vi "N Gaussians Fit Guess Parameters.vi"(8 "N":i32, 9 "Cursor X Array":dbl[](array[numeric]), 10 "Y Array":dbl[](array[numeric]), 11 "X Array":dbl[](array[numeric])) -> (1 "Guess Parameters Array":dbl[](array[numeric]), 2 "Y Array dup":dbl[](array[numeric]), 3 "X Array dup":dbl[](array[numeric]))   [LabVIEW 2019]
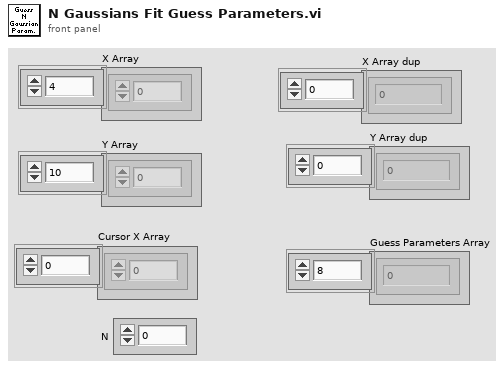
[diagram p1: front panel]
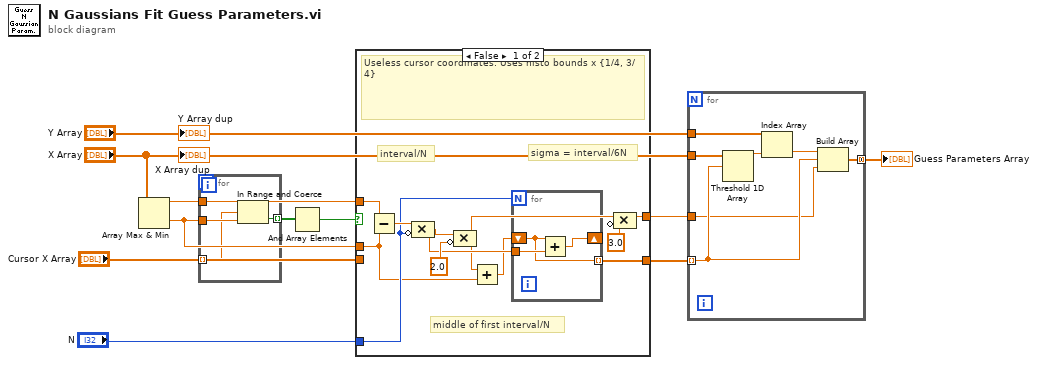
[diagram p0: block diagram]
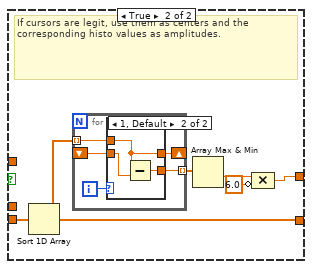
[diagram p2: hidden frame]
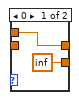
[diagram p3: hidden frame]
diagram:
  n1 = Array Max & Min(array="X Array") -> (max value=w4:dbl, min value=w3:dbl)  [unwired: 2 out]
  n2 = for {
    tunnel: w4 -> [w15]
    tunnel: w3 -> [w14]
    tunnel: "Cursor X Array" -> [w13] mode=indexing
    tunnel: [w12] -> w9 mode=indexing
    n3 = In Range and Coerce(upper limit=w15, x=w13, lower limit=w14) -> (In Range?=w12:bool)  [unwired: 1 out]
  }
  n4 = And Array Elements(Boolean array=w9) -> (logical AND=w1:bool)
  n5 = case shown="False" w1 {
    tunnel: "Cursor X Array" -> [_ w35]
    tunnel: [w21 w34] -> w7
    tunnel: [w20 w31] -> w5
    tunnel: w4 -> [w26 _]
    tunnel: w3 -> [w17 _]
    tunnel: "N" -> [w23 _]
    frame False {
      # "sigma = interval/6N"
      # "middle of first interval/N"
      # "interval/N"
      # "Useless cursor coordinates. Uses histo bounds x {1/4, 3/4}"
      n6 = Subtract(x=w26, y=w17) -> (x-y=w25:dbl)
      n7 = Compound Arithmetic op=MULTIPLY(w25, invert w23) -> (w22:dbl)
      n8 = Compound Arithmetic op=MULTIPLY(w22, invert 2.0 ("value")) -> (w18:dbl)
      n9 = Add(x=w18, y=w17) -> (x+y=w16:dbl)
      n10 = for {
        N: w23 -> [_]
        shift-right: [w29] -> _
        shift-left: w16 -> [w27]
        tunnel: w22 -> [w28]
        tunnel: [w27] -> w21 mode=indexing
        n11 = Add(x=w27, y=w28) -> (x+y=w29:dbl)
      }
      n12 = Compound Arithmetic op=MULTIPLY(w18, invert 3.0 ("value")) -> (w20:dbl)
    }
    frame True {
      # "If cursors are legit, use them as centers and the corresponding histo values as amplitudes."
      n13 = Sort 1D Array(array=w35) -> (sorted array=w34:dbl[])
      n14 = for {
        tunnel: w34 -> [w38] mode=indexing
        shift-right: [w39] -> _
        shift-left: _ -> [w37]
        tunnel: [w36] -> w33 mode=indexing
        i -> [w40]
        n15 = case shown="1, Default" w40 {
          tunnel: [w42 w44] -> w39
          tunnel: w38 -> [w42 w44]
          tunnel: w37 -> [_ w45]
          tunnel: [inf w43] -> w36
          frame 0 {
          }
          frame 1, Default {
            n16 = Subtract(x=w44, y=w45) -> (x-y=w43:dbl)
          }
        }
      }
      n17 = Array Max & Min(array=w33) -> (min value=w32:dbl)  [unwired: 3 out]
      n18 = Compound Arithmetic op=MULTIPLY(w32, invert 6.0 ("value")) -> (w31:dbl)
    }
  }
  n19 = for {
    tunnel: "X Array" -> [w51]
    tunnel: "Y Array" -> [w50]
    tunnel: w7 -> [w48] mode=indexing
    tunnel: [w47] -> w6 mode=concatenating
    tunnel: w5 -> [w46]
    n20 = Threshold 1D Array(2:w48, 3:w51) -> (0:w52:dbl)  [unwired: 1 in]
    n21 = Index Array(array=w50, index=w52) -> (element=w49:dbl)
    n22 = Build Array(w49, w48, w46) -> (w47:dbl[])
  }
  "Guess Parameters Array" <- w6
  "X Array dup" <- "X Array"
  "Y Array dup" <- "Y Array"
